vi "TagDB-IsValid.vi"(8 "error in (no error)":errorcluster, 11 "TagDB":T1) -> (0 "error out":errorcluster, 2 "valid TagDB?":bool, 3 "TagDB(dup)":T1)   [LabVIEW 2017, in "TagDB.lvlib"]
uses:
  TagDB.lvlib
  Typedef/TagDB.ctl
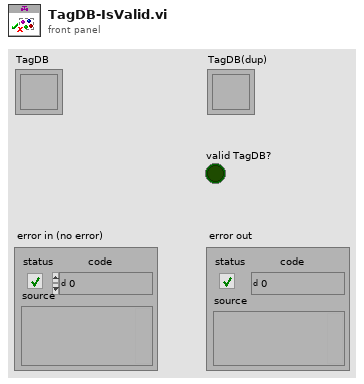
[diagram p1: front panel]
types:
  T1 = typedef "TagDB.lvlib/TagDB.ctl" = refnum<k1>
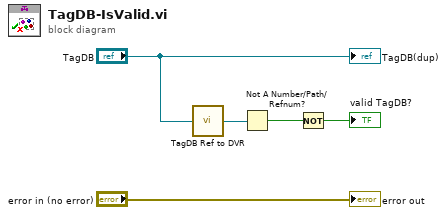
[diagram p0: block diagram]
diagram:
  n1 = call "TagDB Ref to DVR.vi"("TagDB"="TagDB") -> ("DVR"=w3:refnum<data-value>)  [unwired: 4 in]
  n2 = Not A Number/Path/Refnum?(number/path/refnum=w3) -> (NaN/Path/Refnum?=w2:bool)
  n3 = Not(x=w2) -> (.not. x?=→"valid TagDB?":bool)
  "error out" <- "error in (no error)"
  "TagDB(dup)" <- "TagDB"
